vi "FrozenFraction_Extraction.vi"(9 "Sorted Freeze Idx / Part > idx":i32[](array[numeric]), 10 "Sorted Freeze / Part > idx":dbl[][](array[numeric]), 11 "MaxSize":i32) -> (1 "FroozenFraction Graph":dbl[](array[numeric]), 3 "Freeze Fraction":dbl[](array[numeric]))   [LabVIEW 2022 SP3]
uses:
  0069657a-d384-470d-9c09-99f5229114b3.vi
  72d7d6fb-5b23-4d24-8d1e-f3fe31070dd2.vi
  <vilib>/Comparison/Less/Less Functor/Less Functor.lvclass
panel:
  out "sorted idx > freeze fractc > freeze idx":dbl[][](array[numeric])
  out "Sorted Freeze / Part > idx 2":dbl[][](array[numeric])
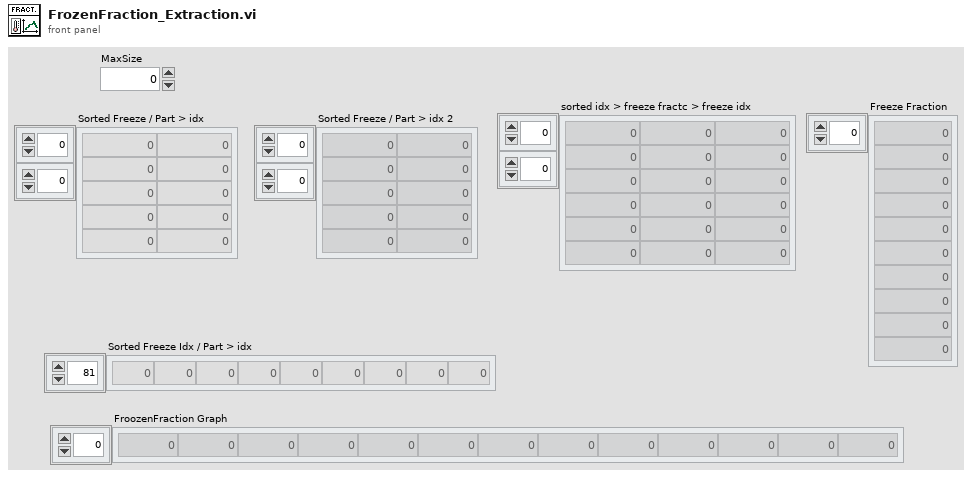
[diagram p1: front panel]
types:
  T1 = cluster{"Sorted Freeze / Part > idx[0]":dbl, "Sorted Freeze / Part > idx[1]":dbl, "Sorted Freeze / Part > idx[2]":dbl, "Sorted Freeze / Part > idx[3]":dbl, "Sorted Freeze / Part > idx[4]":dbl, "Sorted Freeze / Part > idx[5]":dbl, "Sorted Freeze / Part > idx[6]":dbl, "Sorted Freeze / Part > idx[7]":dbl, "Sorted Freeze / Part > idx[8]":dbl}
  T2 = cluster{"Sorted Freeze / Part > idx[0]":dbl, "Sorted Freeze / Part > idx[1]":dbl, "Sorted Freeze / Part > idx[2]":dbl, "Sorted Freeze / Part > idx[3]":dbl, "Sorted Freeze / Part > idx[4]":dbl, "Sorted Freeze / Part > idx[5]":dbl, "Sorted Freeze / Part > idx[6]":dbl, "Sorted Freeze / Part > idx[7]":dbl, "Sorted Freeze / Part > idx[8]":dbl}[]
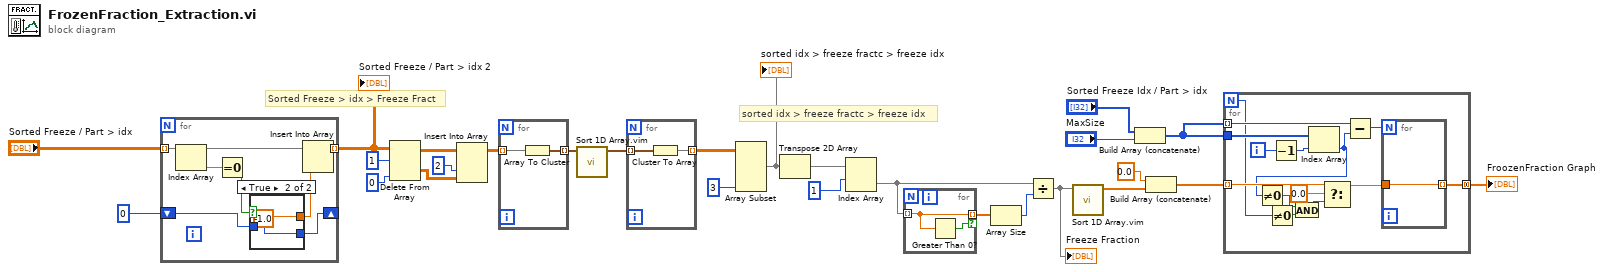
[diagram p0: block diagram]
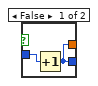
[diagram p2: hidden frame]
diagram:
  # "sorted idx > freeze fractc > freeze idx"
  # "Sorted Freeze > idx > Freeze Fract"
  n1 = for {
    tunnel: "Sorted Freeze / Part > idx" -> [w33] mode=indexing
    tunnel: [w34] -> w14 mode=indexing
    shift-right: [w28] -> _
    shift-left: 0 -> [w29]
    n2 = Index Array(array=w33) -> (element=w32:dbl)  [unwired: 1 in]
    n3 = Equal To 0?(x=w32) -> (x = 0?=w31:bool)
    n4 = case shown="True" w31 {
      tunnel: [w35 -1.0] -> w30
      tunnel: w29 -> [w36 w38]
      tunnel: [w35 w38] -> w28
      frame False {
        n5 = Increment(x=w36) -> (x+1=w35:i32)
      }
      frame True {
      }
    }
    n6 = Insert Into Array(array=w33, new element=w30) -> (w34:dbl[])  [unwired: 1 in]
  }
  "Sorted Freeze / Part > idx 2" <- w14
  n7 = Delete From Array(array=w14, length=1, index (col)=0 ("disabled index (col)")) -> (deleted portion=w22:dbl[][], array with subset deleted=w17:dbl[][])  [unwired: 1 in]
  n8 = Insert Into Array(array=w17, index (col)=2 ("disabled index (col)"), new element=w22) -> (w20:dbl[][])  [unwired: 1 in]
  n9 = for {
    tunnel: w20 -> [w40] mode=indexing
    tunnel: [w39] -> w18 mode=indexing
    n10 = Array To Cluster(array=w40) -> (cluster=w39:T1)
  }
  n11 = call "Sort 1D Array.vim"("unsorted array"=w18) -> ("sorted array"=w6:T2)  [unwired: 10 in]
  n12 = for {
    tunnel: w6 -> [w42] mode=indexing
    tunnel: [w41] -> w19 mode=indexing
    n13 = Cluster To Array(cluster=w42) -> (array=w41:dbl[])
  }
  n14 = Array Subset(array=w19, length (col)=3 ("length")) -> (w5:dbl[][])  [unwired: 3 in]
  "sorted idx > freeze fractc > freeze idx" <- w5
  n15 = Transpose 2D Array(2D array=w5) -> (transposed array=w25:dbl[][])
  n16 = Index Array(array=w25, index (row)=1) -> (element=w2:dbl[])  [unwired: 1 in]
  n17 = for {
    tunnel: w2 -> [w44] mode=indexing
    tunnel: [w44] -> w1 mode=indexing if=w43
    n18 = Greater Than 0?(x=w44) -> (x > 0?=w43:bool)
  }
  n19 = Array Size(array=w1) -> (size(s)=w4:i32)
  n20 = Divide(x=w2, y=w4) -> (x/y=w10:dbl[])
  "Freeze Fraction" <- w10
  n21 = call "Sort 1D Array.vim"("unsorted array"=w10) -> ("sorted array"=w9:dbl[])  [unwired: 10 in]
  n22 = Build Array (concatenate)("Sorted Freeze Idx / Part > idx", "MaxSize") -> (w12:i32[])
  n23 = Build Array (concatenate)(0.0, w9) -> (w11:dbl[])
  n24 = for {
    N -> [w48]
    tunnel: w11 -> [w57] mode=indexing
    tunnel: w12 -> [w58] mode=indexing
    tunnel: [w52] -> w8 mode=concatenating
    tunnel: w12 -> [w56]
    i -> [w55]
    n25 = Not Equal To 0?(x=w48) -> (x != 0?=w50:bool)
    n26 = Decrement(x=w55) -> (x-1=w54:i32)
    n27 = Index Array(array=w56, index=w54) -> (element=w45:i32)
    n28 = Not Equal To 0?(x=w45) -> (x != 0?=w46:bool)
    n29 = And(x=w46, y=w50) -> (x .and. y?=w49:bool)
    n30 = Select(t=w57, s=w49, f=0.0) -> (s? t:f=w51:dbl)
    n31 = Subtract(x=w58, y=w45) -> (x-y=w53:i32)
    n32 = for {
      N: w53 -> [_]
      tunnel: w51 -> [w59]
      tunnel: [w59] -> w52 mode=indexing
    }
  }
  "FroozenFraction Graph" <- w8
